vi "문자열 배열 차원변경_TEST.vi"() -> ()   [LabVIEW 2023]
panel:
  out "출력 배열":string[][](array[string])
  out "전치된 배열":string[][](array[string])
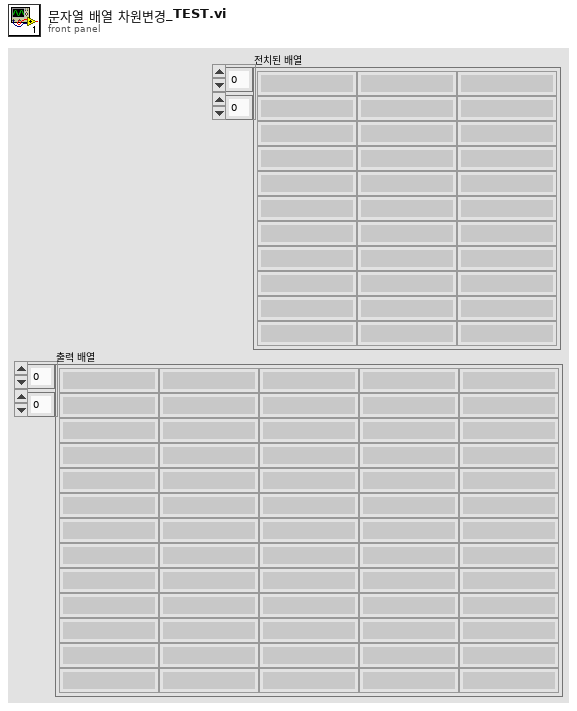
[diagram p1: front panel]
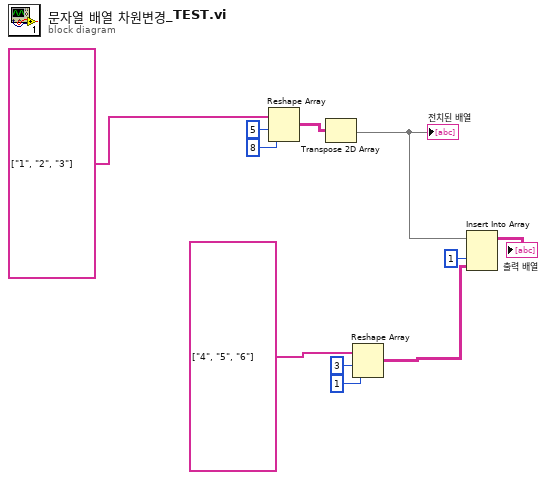
[diagram p0: block diagram]
diagram:
  n1 = Reshape Array(string[] ["1", "2", "3"], 5 ("차원 크기"), 8 ("차원 크기")) -> (w8:string[][])
  n2 = Transpose 2D Array(2D array=w8) -> (transposed array=w7:string[][])
  "전치된 배열" <- w7
  n3 = Reshape Array(string[] ["4", "5", "6"], 3 ("차원 크기"), 1 ("차원 크기")) -> (w1:string[][])
  n4 = Insert Into Array(array=w7, index (col)=1 ("비활성화된 인덱스 (열)"), new element=w1) -> (→"출력 배열":string[][])  [unwired: 1 in]
